vi "Get Source.vi"(8 "error in (no error)":errorcluster, 11 "NMEA Message in":refnum<class "NMEA Message.lvclass">) -> (0 "error out":errorcluster, 2 "Source":string, 3 "NMEA Message out":refnum<class "NMEA Message.lvclass">)   [LabVIEW 2020, in "nmea.lvlib" / "NMEA Message.lvclass"]
uses:
  NMEA Message.lvclass
  NMEA Message.lvclass/NMEA Message.ctl
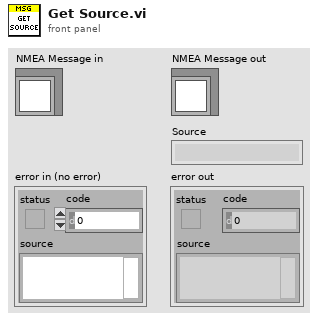
[diagram p1: front panel]
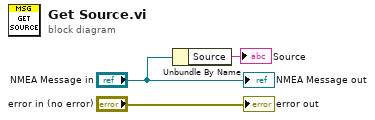
[diagram p0: block diagram]
diagram:
  n1 = Unbundle By Name("NMEA Message in") -> ("Source"=→"Source":string)
  "error out" <- "error in (no error)"
  "NMEA Message out" <- "NMEA Message in"
